vi "sub_post_and_clear_error.vi"(8 "error in (no error)":errorcluster, 10 "Post Error Status":bool, 11 "daq.io type in":T1={"daq.io ref"=refnum, "daq.io API Base"="http://dashboard.daq.io/api/v1", "Device Key"="DESKTOP_7UDDDR9_LOCALDOMAIN_TYPE", "Account ID"="DESKTOP_7UDDDR9_LOCALDOMAIN", "online"=TRUE, "SSL"=TRUE, "buffer"=TRUE}) -> (0 "error out":errorcluster, 3 "daq.io type out":T1={"daq.io ref"=refnum, "daq.io API Base"="", "Device Key"="", "Account ID"="", "online"=TRUE, "SSL"=FALSE, "buffer"=TRUE})   [LabVIEW 2013, in "daqio minimal.lvlib"]
doc: "This VI posts or buffers an occuring error event to the System Status Event route and clears the error."
uses:
  daqio minimal.lvlib
  _typedefs/daqio-Type.ctl
  <vilib>/httpClient/ClientHandle.ctl
  <vilib>/httpClient/LabVIEWHTTPClient.lvlib
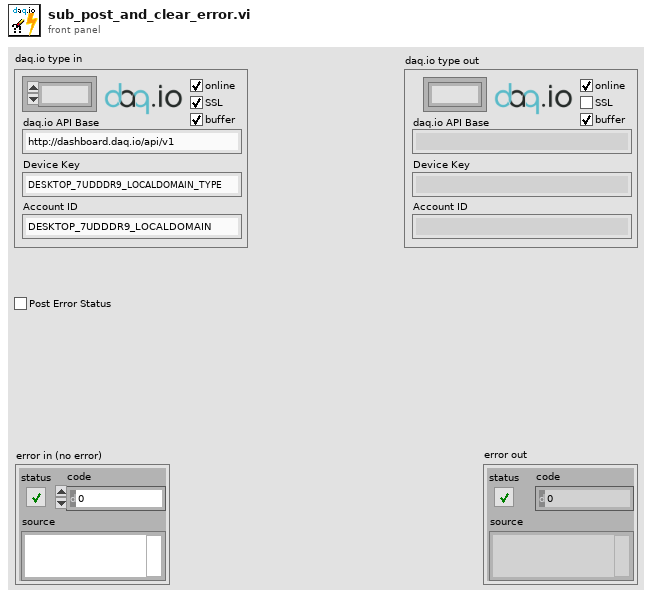
[diagram p1: front panel]
types:
  T1 = typedef "daqio minimal.lvlib/daqio-Type.ctl" = cluster{"daq.io ref":T2, "daq.io API Base":string, "Device Key":string, "Account ID":string, "online":bool, "SSL":bool, "buffer":bool}
  T2 = typedef "LabVIEWHTTPClient.lvlib/ClientHandle.ctl" = refnum<k1>
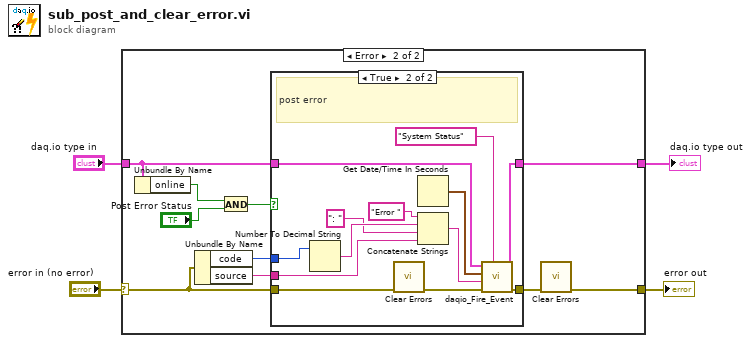
[diagram p0: block diagram]
diagram:
  n1 = case shown="Error" "error in (no error)" {
    selector: "error in (no error)" -> [w5 w11]
    tunnel: "daq.io type in" -> [w6 w10]
    tunnel: [w6 w16] -> w2
    tunnel: [w5 w12] -> w1
    frame No Error {
    }
    frame Error {
      n2 = Unbundle By Name(w10) -> ("online"=w8:bool)
      n3 = Unbundle By Name(w11) -> ("code"=w15:i32, "source"=w14:string)
      n4 = And(x=w8, y="Post Error Status") -> (x .and. y?=w9:bool)
      n5 = case shown="True" w9 {
        tunnel: w10 -> [w17 w30]
        tunnel: [w17 w29] -> w16
        tunnel: w15 -> [_ w27]
        tunnel: w14 -> [_ w23]
        tunnel: [w18 w21] -> w13
        tunnel: w11 -> [w18 w20]
        frame False {
          # "don't post error message (default) when offline"
        }
        frame True {
          # "post error"
          n6 = Number To Decimal String(number=w27) -> (decimal integer string=w25:string)  [unwired: 1 in]
          n7 = call <vilib>:"Clear Errors.vi"("error in (no error)"=w20) -> ("error out"=w19:errorcluster)  [unwired: 6 in]
          n8 = Get Date/Time In Seconds() -> (seconds since 1Jan1904=w31:timestamp)
          n9 = Concatenate Strings("Error " ("string"), w25, ": " ("string"), w23) -> (w22:string)
          n10 = call "daqio_Fire_Event.vi"("Event Key"="System Status", "error in (no error)"=w19, "Event Value"=w22, "Event Date and Time"=w31, "daq.io type in"=w30) -> ("error out"=w21:errorcluster, "daq.io type out"=w29:T1)  [unwired: 5 in]
        }
      }
      n11 = call <vilib>:"Clear Errors.vi"("error in (no error)"=w13) -> ("error out"=w12:errorcluster)  [unwired: 6 in]
    }
  }
  "daq.io type out" <- w2
  "error out" <- w1
